vi "Test - Add to Definition.vi"   [LabVIEW 2023, in "JSON Schema Generator.lvlib"]
uses:
  JSON Schema Generator.lvlib
  Defintion FGV Actions.ctl
  <vilib>/addons/_JKI Toolkits/Caraya/classes/Assert/Assert Equal Value_Variant.vi
  <vilib>/addons/_JKI Toolkits/Caraya/classes/Assert/Assert Not Error.vi
  <vilib>/addons/_JKI Toolkits/Caraya/classes/Test/Test.lvclass
  <vilib>/addons/_JKI Toolkits/Caraya/classes/Assert/Assert.lvclass
types:
  T1 = typedef "JSON Schema Generator.lvlib/Defintion FGV Actions.ctl" = enum16{"Create Defs", "Update Defs", "Get all Defs", "Get Def"}
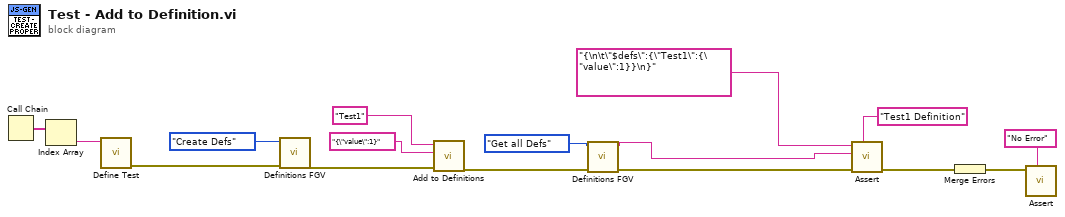
[diagram p0: block diagram]
diagram:
  n1 = Call Chain() -> (call chain=w16:string[])
  n2 = Index Array(array=w16) -> (element=w15:string)  [unwired: 1 in]
  n3 = call <vilib>:"Define Test.vi"("Label (VI Title)"=w15) -> ("error out"=w3:errorcluster)  [unwired: 9 in, 1 out]
  n4 = call "Definitions FGV.vi"("error in (no error)"=w3, "Action"=Defintion_FGV_Actions."Create Defs") -> ("error out"=w2:errorcluster)  [unwired: 7 in, 2 out]
  n5 = call "Add to Definitions.vi"("error in (no error)"=w2, "Definition Schema"="{\"value\":1}", "Name"="Test1") -> ("error out"=w1:errorcluster)  [unwired: 8 in]
  n6 = call "Definitions FGV.vi"("error in (no error)"=w1, "Action"=Defintion_FGV_Actions."Get all Defs") -> ("error out"=w9:errorcluster, "Definitions out"=w7:string)  [unwired: 7 in, 1 out]
  n7 = call-poly <vilib>:"Assert.vi"("Label"="Test1 Definition", "error in (no error)"=w9, "Y"=w7, "X"="{\n\t\"$defs\":{\"Test1\":{\"value\":1}}\n}") -> ("error out"=w13:errorcluster)  [unwired: 6 in, 1 out]
  n8 = Merge Errors(w13) -> (w11:errorcluster)
  n9 = call-poly <vilib>:"Assert.vi"("Label"="No Error", "Not Error?"=w11) -> ()  [unwired: 8 in, 2 out]
